vi "Periodic Tasks.vi"(8 "error in (no error)":errorcluster) -> ()   [LabVIEW 2011]
doc: "This VI runs in parallel to other tasks. It can contain as many user-defined periodic loops as you need. These can carry out PID or other sorts of timed response."
uses:
  <vilib>/Rock Robotics/SystemInterfaces/Utilities/FPGA_UtilitiesLED State.ctl
  <vilib>/Rock Robotics/SystemInterfaces/Utilities/FPGA_UtilitiesLED Source.ctl
  Robot Global Data.vi
  <vilib>/Rock Robotics/WPI/Compressor/WPI_CompressorGetSetRefNum.vi
panel:
  out "At Speed":bool
  in  "Spin Time (ms)":u32=400
  in  "Shooter Th (RPM)":dbl=300.0
  out "Shot Sensor":bool
  in  "Squish TH 2":dbl=4.0
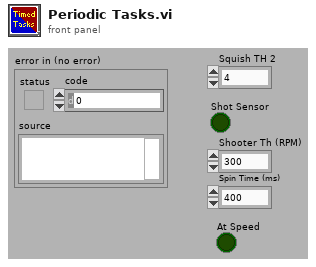
[diagram p1: front panel]
types:
  T1 = typedef "WPI_AnalogChannelDevRef.ctl" = cluster{"DevStatus":errorcluster, "Analog Module":T2, "Analog Channel":T3}
  T2 = typedef "FPGA_TypedefAnalogModule.ctl" = enum16{"Analog Module 1", "Analog Module 2"}
  T3 = typedef "FPGA_AIChannel.ctl" = enum8{"AI 1", "AI 2", "AI 3", "AI 4", "AI 5", "AI 6", "AI 7", "AI 8", "Invalid"}
  T4 = typedef "WPI_EncoderDevRef.ctl" = cluster{"DevStatus":errorcluster, "EncoderIndex":T5, "CounterIndex":T6, "DistancePerCount":dbl, "Decoding Type":T7}
  T5 = typedef "FPGA_EncoderIdx.ctl" = enum8{"Enc 0", "Enc 1", "Enc 2", "Enc 3", "Invalid"}
  T6 = typedef "FPGA_CounterCtrSystemIndex.ctl" = enum8{"Ctr 0", "Ctr 1", "Ctr 2", "Ctr 3", "Ctr 4", "Ctr 5", "Ctr 6", "Ctr 7", "Invalid"}
  T7 = typedef "WPI_EncoderType.ctl" = enum16{"1x", "2x", "4x"}
  T8 = typedef "Semaphore RefNum" = refnum<k1>
  T9 = typedef "WPI_MotorControlDeviceRef.ctl" = cluster{"DeviceStatus":errorcluster, "Type":enum16{"PWM", "CAN"}, "PWM":cluster{"Digital Module":T10, "PWM Channel":T11, "DeadBand":T12}, "CAN":cluster{"Device Number":u8, "Control Mode":T13, "Semaphore":T8, "Max Vout":dbl}, "Invert":bool, "TransformRef":T14, "InvTransformRef":T14}
  T10 = typedef "FPGA_TypedefDigitalModule.ctl" = enum16{"Digital Module 1", "Digital Module 2"}
  T11 = typedef "FPGA_DIOPWMChannel.ctl" = enum8{"PWM 1", "PWM 2", "PWM 3", "PWM 4", "PWM 5", "PWM 6", "PWM 7", "PWM 8", "PWM 9", "PWM 10", "Invalid"}
  T12 = typedef "WPI_PWMDeadband.ctl" = cluster{"Name":string, "maxPositivePwm":i32, "minPositivePwm":i32, "centerPwm":i32, "maxNegativePwm":i32, "minNegativePwm":i32, "angularRange":u16}
  T13 = typedef "WPI_CANJaguar_ControlMode.ctl" = enum8{"Percent VBus", "Current", "Speed", "Position", "Voltage"}
  T14 = typedef "WPI_PWMTransform_ConPane.ctl" = refnum<vi>
  T15 = typedef "WPI_DigitalInputDevRef.ctl" = cluster{"DevStatus":errorcluster, "DIO Channel":T16, "Digital Module":T10}
  T16 = typedef "FPGA_DIOChannel.ctl" = enum8{"DIO 1", "DIO 2", "DIO 3", "DIO 4", "DIO 5", "DIO 6", "DIO 7", "DIO 8", "DIO 9", "DIO 10", "DIO 11", "DIO 12", "DIO 13", "DIO 14", "Invalid"}
  T17 = typedef "ShooterData.ctl" = cluster{"Setpoint":dbl, "Speed":dbl, "Squish":dbl, "Shot Sensor":bool, "At Speed":bool}
  T18 = typedef "Target Typedef.ctl" = cluster{"X":dbl, "Y":dbl, "Deltax":dbl, "Distance":dbl}
  T19 = typedef "Autonomous Data.ctl" = cluster{"Auto Mode":enum16{"Do Nothing", "Shoot From Key", "Shoot From Key Center, Bridge", "Shoot From Key, Feed", "Shoot From Key, Drive Forward", "Fender From Center", "Fender From Right", "Fender From Left"}, "Delay (s)":dbl}
  T20 = typedef "FPGA_UtilitiesLED State.ctl" = enum16{"Off", "On", "Toggle"}
  T21 = typedef "FPGA_UtilitiesLED Source.ctl" = enum16{"User LED", "FPGA LED"}
  T22 = typedef "WPI_CompressorDevRef.ctl" = cluster{"DevStatus":errorcluster, "DigitalInputDevRef":T15, "RelayDevRef":T23}
  T23 = typedef "WPI_RelayDevRef.ctl" = cluster{"DevStatus":errorcluster, "Relay Channel":T24, "Digital Module":T10, "Relay Direction":T25}
  T24 = typedef "FPGA_DIORelayChannel.ctl" = enum8{"Relay 1", "Relay 2", "Relay 3", "Relay 4", "Relay 5", "Relay 6", "Relay 7", "Relay 8", "Invalid"}
  T25 = typedef "WPI_RelayDirection.ctl" = enum16{"Both directions", "Forward only", "Reverse only"}
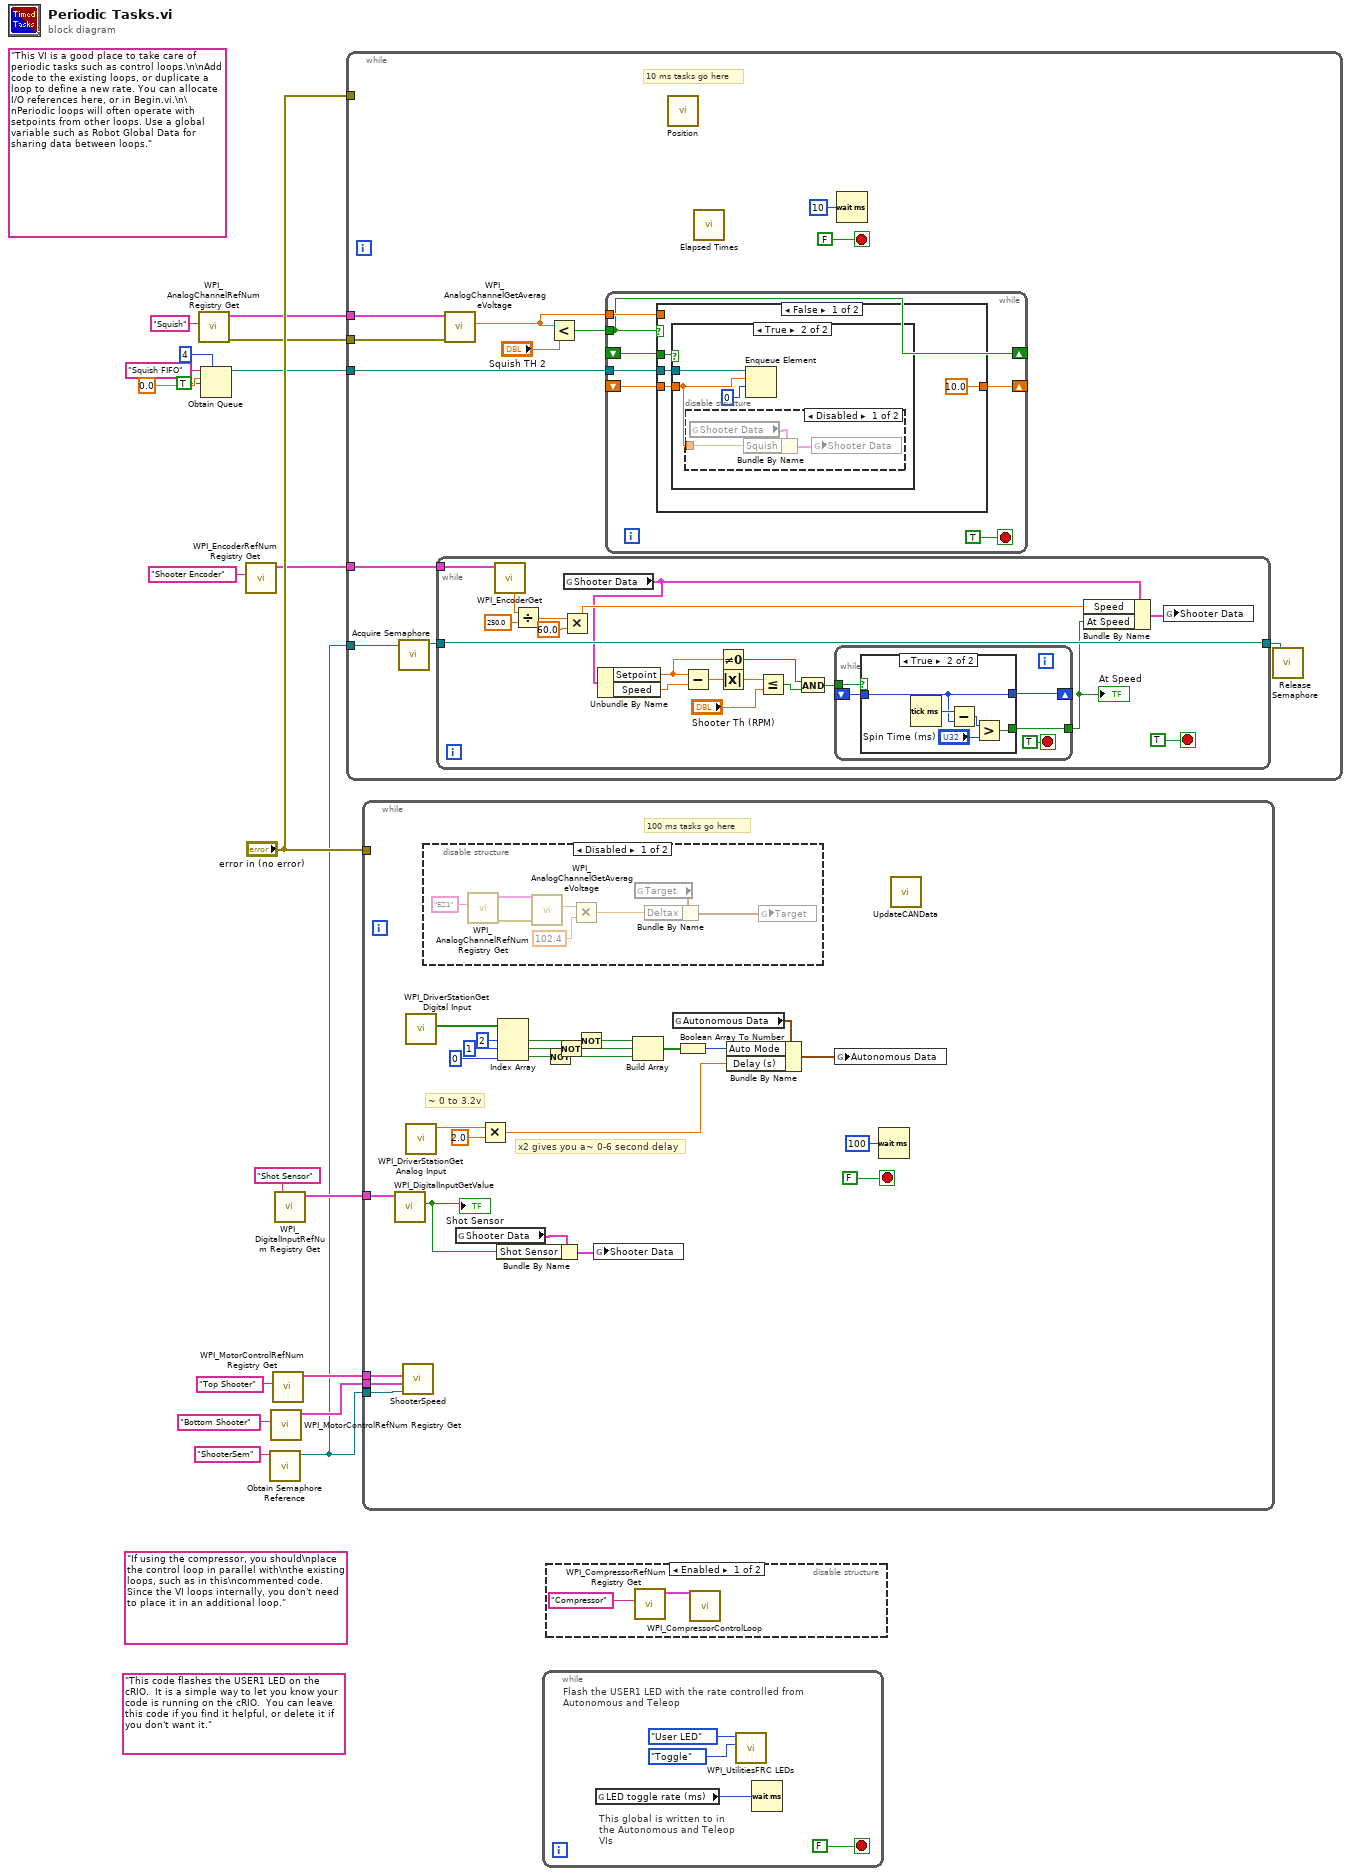
[diagram p0: block diagram]
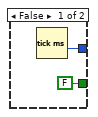
[diagram p4: hidden frame]
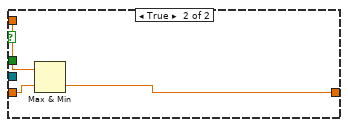
[diagram p7: hidden frame]
diagram:
  (unwired) "If using the compressor, you should\nplace the control loop in parallel with\nthe existing loops, such as in this\ncommented code. Since the VI loops internally, you don't need to place it in an additional loop."
  (unwired) "This code flashes the USER1 LED on the cRIO.  It is a simple way to let you know your code is running on the cRIO.  You can leave this code if you find it helpful, or delete it if you don't want it."
  (unwired) "This VI is a good place to take care of periodic tasks such as control loops.\n\nAdd code to the existing loops, or duplicate a loop to define a new rate. You can allocate I/O references here, or in Begin.vi.\n\nPeriodic loops will often operate with setpoints from other loops. Use a global variable such as Robot Global Data for sharing data between loops."
  n1 = call <vilib>:"WPI_AnalogChannelRefNum Registry Get.vi"("refnum name"="Squish") -> ("error out"=w12:errorcluster, "AIDeviceRef"=w13:T1)  [unwired: 9 in]
  n2 = Obtain Queue(max queue size (-1, unlimited)=4, name (unnamed)="Squish FIFO", element data type=sgl 0.0 ("Voltage"), create if not found? (T)=TRUE) -> (queue out=w11:refnum<queue>)  [unwired: 1 in, 2 out]
  n3 = call <vilib>:"WPI_EncoderRefNum Registry Get.vi"("refnum name"="Shooter Encoder") -> ("EncoderDevRef"=w2:T4)  [unwired: 9 in, 1 out]
  n4 = call <vilib>:"Obtain Semaphore Reference.vi"("name (unnamed)"="ShooterSem") -> ("semaphore"=w1:T8)  [unwired: 4 in, 2 out]
  n5 = call <vilib>:"WPI_MotorControlRefNum Registry Get.vi"("refnum name"="Bottom Shooter") -> ("MotorControlDevRef"=w3:T9)  [unwired: 9 in, 1 out]
  n6 = call <vilib>:"WPI_MotorControlRefNum Registry Get.vi"("refnum name"="Top Shooter") -> ("MotorControlDevRef"=w4:T9)  [unwired: 9 in, 1 out]
  n7 = call <vilib>:"WPI_DigitalInputRefNum Registry Get.vi"("refnum name"="Shot Sensor") -> ("DigitalInputDevRef"=w5:T15)  [unwired: 9 in, 1 out]
  n8 = while {
    tunnel: "error in (no error)" -> [_]
    tunnel: w13 -> [w26]
    tunnel: w12 -> [w25]
    tunnel: w11 -> [w24]
    tunnel: w2 -> [w23]
    tunnel: w1 -> [w22]
    stop <- FALSE stop-if-true
    # "10 ms tasks go here"
    n9 = call <vilib>:"Acquire Semaphore.vi"("semaphore"=w22) -> ("semaphore out"=w21:T8)  [unwired: 4 in, 2 out]
    n10 = while {
      tunnel: w23 -> [w44]
      tunnel: w21 -> [w42]
      tunnel: [w42] -> w20
      stop <- TRUE stop-if-true
      n11 = call <vilib>:"WPI_EncoderGet.vi"("EncoderDevRef"=w44) -> ("Rate"=w48:dbl)  [unwired: 5 in, 5 out]
      n12 = Divide(x=w48, y=250.0) -> (x/y=w47:dbl)
      n13 = Multiply(x=w47, y=60.0) -> (x*y=w45:dbl)
      n14 = global read "Robot Global Data.vi" "Shooter Data"() -> (w37:T17)
      n15 = Unbundle By Name(w37) -> ("Setpoint"=w35:dbl, "Speed"=w38:dbl)
      n16 = Subtract(x=w35, y=w38) -> (x-y=w39:dbl)
      n17 = Not Equal To 0?(x=w35) -> (x != 0?=w33:bool)
      n18 = Absolute Value(x=w39) -> (abs(x)=w40:dbl)
      n19 = Less Or Equal?(x=w40, y="Shooter Th (RPM)") -> (x <= y?=w34:bool)
      n20 = And(x=w33, y=w34) -> (x .and. y?=w32:bool)
      n21 = while {
        tunnel: w32 -> [w55]
        shift-right: [w53] -> _
        shift-left: _ -> [w51]
        tunnel: [w52] -> w36
        stop <- TRUE stop-if-true
        n22 = case shown="True" w55 {
          tunnel: [w57 w61] -> w53
          tunnel: [FALSE ("Shot") w60] -> w52
          tunnel: w51 -> [_ w61]
          frame False {
            n23 = Tick Count (ms)() -> (millisecond timer value=w57:u32)
          }
          frame True {
            n24 = Tick Count (ms)() -> (millisecond timer value=w62:u32)
            n25 = Subtract(x=w62, y=w61) -> (x-y=w59:u32)
            n26 = Greater?(x=w59, y="Spin Time (ms)") -> (0:w60:bool)
          }
        }
      }
      "At Speed" <- w36
      n27 = Bundle By Name(cluster=w37, "Speed"=w45, "At Speed"=w36) -> (w50:T17)
      n28 = global write "Robot Global Data.vi" "Shooter Data"(w50) -> ()
    }
    n29 = call <vilib>:"WPI_AnalogChannelGetAverageVoltage.vi"("error in (no error)"=w25, "AIDeviceRef"=w26) -> ("Voltage"=w27:dbl)  [unwired: 7 in, 2 out]
    n30 = Less?(x=w27, y="Squish TH 2") -> (x < y?=w28:bool)
    n31 = while {
      tunnel: w28 -> [w65]
      tunnel: w27 -> [w68]
      shift-right: [w67] -> _
      shift-left: _ -> [w66]
      shift-right: [w65] -> _
      shift-left: _ -> [w64]
      tunnel: w24 -> [w63]
      stop <- TRUE stop-if-true
      n32 = case shown="False" w65 {
        tunnel: w68 -> [_ w81]
        tunnel: [sgl 10.0 ("Voltage") w80] -> w67
        tunnel: w66 -> [w71 w82]
        tunnel: w64 -> [w72 _]
        tunnel: w63 -> [w70 _]
        frame False {
          n33 = case shown="True" w72 {
            tunnel: w71 -> [_ w74]
            tunnel: w70 -> [_ w76]
            frame False {
            }
            frame True {
              n34 = disable-structure shown="Disabled" {
                disable-tunnel: w74 -> [w77 _]
                frame Disabled {
                  n35 = global read "Robot Global Data.vi" "Shooter Data"() -> (w78:T17)
                  n36 = Bundle By Name(cluster=w78, "Squish"=w77) -> (w79:T17)
                  n37 = global write "Robot Global Data.vi" "Shooter Data"(w79) -> ()
                }
                frame Enabled {
                }
              }
              n38 = Enqueue Element(queue=w76, element=w74, timeout in ms (-1)=0) -> ()  [unwired: 1 in, 3 out]
            }
          }
        }
        frame True {
          n39 = Max & Min(x=w81, y=w82) -> (min(x,y)=w80:dbl)  [unwired: 1 out]
        }
      }
    }
    n40 = call "Position.vi"() -> ()  [unwired: 12 in]
    n41 = call "Elapsed Times.vi"() -> ()  [unwired: 3 in, 1 out]
    n42 = Wait (ms)(milliseconds to wait=u32 10) -> ()  [unwired: 1 out]
    n43 = call <vilib>:"Release Semaphore.vi"("semaphore"=w20) -> ()  [unwired: 5 in, 2 out]
  }
  n44 = while {
    tunnel: "error in (no error)" -> [_]
    tunnel: w5 -> [w89]
    tunnel: w4 -> [w85]
    tunnel: w3 -> [w84]
    tunnel: w1 -> [w83]
    stop <- FALSE stop-if-true
    # "~ 0 to 3.2v"
    # "x2 gives you a~ 0-6 second delay"
    # "100 ms tasks go here"
    n45 = call <vilib>:"WPI_DigitalInputGetValue.vi"("DigitalInputDevRef"=w89) -> ("Value"=w86:bool)  [unwired: 8 in, 2 out]
    "Shot Sensor" <- w86
    n46 = call "ShooterSpeed.vi"("semaphore"=w83, "Bottom Shooter"=w84, "Top Shooter"=w85) -> ()  [unwired: 9 in]
    n47 = call <vilib>:"WPI_DriverStationGet Digital Input.vi"() -> ("Driver Station Digital Input (1-8)"=w91:bool[])  [unwired: 11 out]
    n48 = call <vilib>:"WPI_DriverStationGet Analog Input.vi"() -> ("Analog 1 (V)"=w98:dbl)  [unwired: 11 out]
    n49 = disable-structure shown="Disabled" {
      frame Disabled {
        n50 = call <vilib>:"WPI_AnalogChannelRefNum Registry Get.vi"("refnum name"="EZ1") -> ("error out"=w115:errorcluster, "AIDeviceRef"=w114:T1)  [unwired: 9 in]
        n51 = call <vilib>:"WPI_AnalogChannelGetAverageVoltage.vi"("error in (no error)"=w115, "AIDeviceRef"=w114) -> ("Voltage"=w116:dbl)  [unwired: 7 in, 2 out]
        n52 = Multiply(x=w116, y=102.4) -> (x*y=w109:dbl)
        n53 = global read "Robot Global Data.vi" "Target"() -> (w110:T18)
        n54 = Bundle By Name(cluster=w110, "Deltax"=w109) -> (w111:T18)
        n55 = global write "Robot Global Data.vi" "Target"(w111) -> ()
      }
      frame Enabled {
      }
    }
    n56 = global read "Robot Global Data.vi" "Shooter Data"() -> (w87:T17)
    n57 = Multiply(x=w98, y=2.0) -> (x*y=w100:dbl)
    n58 = Bundle By Name(cluster=w87, "Shot Sensor"=w86) -> (w88:T17)
    n59 = Index Array(array=w91, index #1=2 ("index"), index #2=1 ("index"), index #3=0 ("index")) -> (element #1=w104:bool, element #2=w105:bool, element #3=w106:bool)
    n60 = Not(x=w106) -> (.not. x?=w103:bool)
    n61 = Not(x=w105) -> (.not. x?=w102:bool)
    n62 = Not(x=w104) -> (.not. x?=w101:bool)
    n63 = global write "Robot Global Data.vi" "Shooter Data"(w88) -> ()
    n64 = Build Array(w101, w102, w103) -> (w96:bool[])
    n65 = global read "Robot Global Data.vi" "Autonomous Data"() -> (w95:T19)
    n66 = Boolean Array To Number(Boolean array=w96) -> (number=w97:u32)
    n67 = Bundle By Name(cluster=w95, "Auto Mode"=w97, "Delay (s)"=w100) -> (w90:T19)
    n68 = global write "Robot Global Data.vi" "Autonomous Data"(w90) -> ()
    n69 = Wait (ms)(milliseconds to wait=u32 100) -> ()  [unwired: 1 out]
    n70 = call "UpdateCANData.vi"() -> ()  [unwired: 12 in]
  }
  n71 = while {
    stop <- FALSE stop-if-true
    # "This global is written to in the Autonomous and Teleop VIs"
    # "Flash the USER1 LED with the rate controlled from Autonomous and Teleop"
    n72 = global read "Robot Global Data.vi" "LED toggle rate (ms)"() -> (w117:u32)
    n73 = call <vilib>:"WPI_UtilitiesFRC LEDs.vi"("State"=FPGA_UtilitiesLED_State."Toggle", "LED Type"=FPGA_UtilitiesLED_Source."User LED") -> ()  [unwired: 1 in, 9 out]
    n74 = Wait (ms)(milliseconds to wait=w117) -> ()  [unwired: 1 out]
  }
  n75 = disable-structure shown="Enabled" {
    frame Enabled {
      n76 = call <vilib>:"WPI_CompressorRefNum Registry Get.vi"("refnum name"="Compressor") -> ("CompressorDevRef"=w122:T22)  [unwired: 9 in, 1 out]
      n77 = call <vilib>:"WPI_CompressorControlLoop.vi"("CompressorDevRef"=w122) -> ()  [unwired: 11 in]
    }
    frame Disabled {
    }
  }
